vi "to table.vi"(8 "error in":errorcluster, 10 "variant":variant, 11 "configuration in":refnum<class "tag select module configuration.lvclass">) -> (0 "error out":errorcluster, 2 "table":string[][](array[string]), 3 "configuration out":refnum<class "tag select module configuration.lvclass">)   [LabVIEW 2015]
uses:
  <vilib>/NI/Module Execution Interface/Engine Configuration/engine configuration.lvclass
  <vilib>/NI/Tag Bus/tag/tag descriptor.lvclass
  <vilib>/NI/Configuration Framework/serializable configuration/NISE_CEF_serializable configuration.lvclass
  tag select module configuration.lvclass
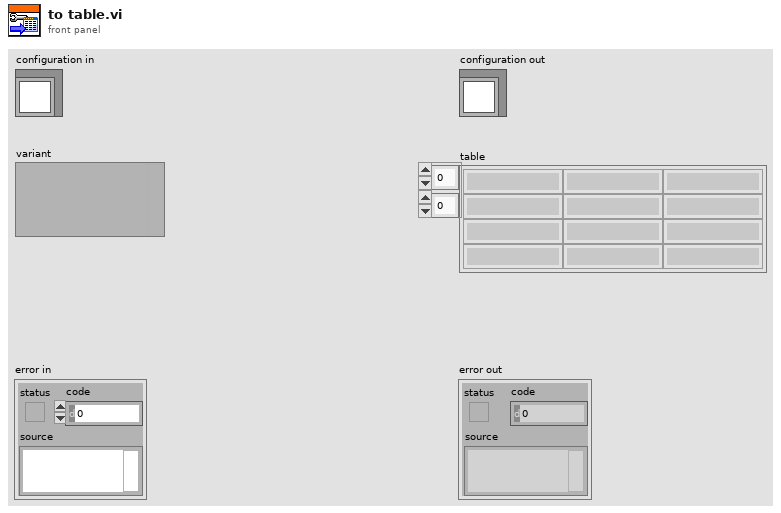
[diagram p1: front panel]
types:
  T1 = typedef "tag select module configuration.lvclass/tag select configuration.ctl" = cluster{"tag select name":string, "data type":T2, "output":refnum<class "TBM channel.lvclass">, "select":refnum<class "TBM channel.lvclass">, "input channels":refnum<class "TBM channel.lvclass">[]}
  T2 = typedef "tag bus.lvlib/tag descriptor.lvclass/Data Type.ctl" = enum16{"Double", "Single", "I64", "I32", "I16", "I8", "U64", "U32", "U16", "U8", "Boolean", "String", "Array of Double", "Array of Single", "Array of I64", "Array of I32", "Array of I16", "Array of I8", "Array of U64", "Array of U32", "Array of U16", "Array of U8", "Array of Boolean", "Array of String"}
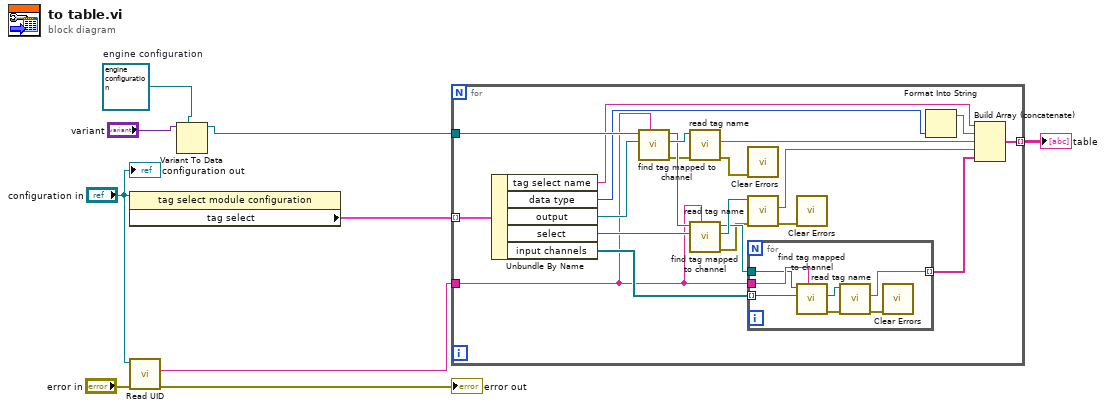
[diagram p0: block diagram]
diagram:
  w1 = refnum<class "engine configuration.lvclass"> refnum  # engine configuration
  n1 = property class="tag select module configuration"(reference="configuration in") -> ("tag select"=w8:T1[])  [unwired: 1 in, 2 out]
  n2 = call <vilib>:"Read UID.vi"("error in"="error in", "configuration in"="configuration in") -> ("error out"=→"error out":errorcluster, "instance id"=w9:string)  [unwired: 7 in, 1 out]
  n3 = Variant To Data(type=w1, Variant="variant") -> (data=w3:refnum<class "engine configuration.lvclass">)  [unwired: 1 in, 1 out]
  n4 = for {
    tunnel: w8 -> [w30] mode=indexing
    tunnel: w3 -> [w29]
    tunnel: w9 -> [w10]
    tunnel: [w17] -> w7 mode=indexing
    n5 = Unbundle By Name(w30) -> ("tag select name"=w21:string, "data type"=w20:T2, "output"=w26:refnum<class "TBM channel.lvclass">, "select"=w25:refnum<class "TBM channel.lvclass">, "input channels"=w27:refnum<class "TBM channel.lvclass">[])
    n6 = call <vilib>:"find tag mapped to channel.vi"("owner"=w10, "channel"=w26, "engine configuration in"=w29) -> ("error out"=w14:errorcluster, "tag"=w28:refnum<class "tag descriptor.lvclass">, "engine configuration out"=w15:refnum<class "engine configuration.lvclass">)  [unwired: 6 in]
    n7 = call <vilib>:"read tag name.vi"("error in"=w14, "system tag in"=w28) -> ("error out"=w11:errorcluster, "name"=w24:string)  [unwired: 7 in, 1 out]
    n8 = call <vilib>:"find tag mapped to channel.vi"("owner"=w10, "channel"=w25, "engine configuration in"=w15) -> ("error out"=w13:errorcluster, "tag"=w23:refnum<class "tag descriptor.lvclass">, "engine configuration out"=w16:refnum<class "engine configuration.lvclass">)  [unwired: 6 in]
    n9 = call <vilib>:"Clear Errors.vi"("error in (no error)"=w11) -> ()  [unwired: 5 in, 2 out]
    n10 = call <vilib>:"read tag name.vi"("error in"=w13, "system tag in"=w23) -> ("error out"=w12:errorcluster, "name"=w22:string)  [unwired: 7 in, 1 out]
    n11 = for {
      tunnel: w10 -> [w37]
      tunnel: w27 -> [w36] mode=indexing
      tunnel: [w34] -> w18 mode=indexing
      tunnel: w16 -> [w33]
      n12 = call <vilib>:"find tag mapped to channel.vi"("owner"=w37, "channel"=w36, "engine configuration in"=w33) -> ("error out"=w32:errorcluster, "tag"=w35:refnum<class "tag descriptor.lvclass">)  [unwired: 6 in, 1 out]
      n13 = call <vilib>:"read tag name.vi"("error in"=w32, "system tag in"=w35) -> ("error out"=w31:errorcluster, "name"=w34:string)  [unwired: 7 in, 1 out]
      n14 = call <vilib>:"Clear Errors.vi"("error in (no error)"=w31) -> ()  [unwired: 5 in, 2 out]
    }
    n15 = call <vilib>:"Clear Errors.vi"("error in (no error)"=w12) -> ()  [unwired: 5 in, 2 out]
    n16 = Format Into String(w20) -> (resulting string=w19:string)  [unwired: 3 in, 1 out]
    n17 = Build Array (concatenate)(w21, w19, w24, w22, w18) -> (w17:string[])
  }
  "table" <- w7
  "configuration out" <- "configuration in"
